vi "read station path config.vi"(8 "error in":errorcluster, 10 "station idx":i32, 11 "configuration file path in":path) -> (0 "error out":errorcluster, 2 "paths":T1={"Base Path"=path "", "system error log path"=path "", "Error Table Path"=path "", "Store errors log path"=path "", "data bytes log path"=path "", "network path"=path "C:/Labview Code/System/Error Table"}, 3 "configuration file path out":path)   [LabVIEW 2018]
uses:
  02.Type Def's/station paths.ctl
  05.UserVI's/file io/ini/type defs/ini file actions.ctl
  05.UserVI's/file io/ini/type defs/ini entry value.ctl
  05.UserVI's/file io/ini/type defs/ini entry types.ctl
  05.UserVI's/file io/ini/type defs/ini entry.ctl
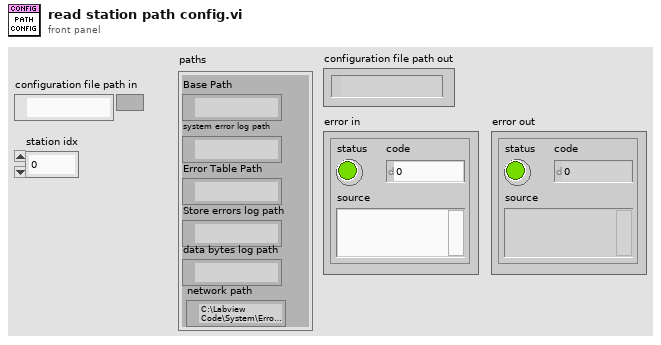
[diagram p1: front panel]
types:
  T1 = typedef "station paths.ctl" = cluster{"Base Path":path, "system error log path":path, "Error Table Path":path, "Store errors log path":path, "data bytes log path":path, "network path":path}
  T2 = typedef "ini entry value.ctl" = cluster{"Boolean":bool, "Dbl":dbl, "I32":i32, "Path":path, "String":string, "U32":u32}
  T3 = typedef "ini file actions.ctl" = enum16{"read ini", "write ini"}
  T4 = typedef "ini entry.ctl" = cluster{"section":string, "key":string, "type":T5, "default value":T2}
  T5 = typedef "ini entry types.ctl" = enum16{"Boolean", "Double", "I32", "Path", "String", "U32"}
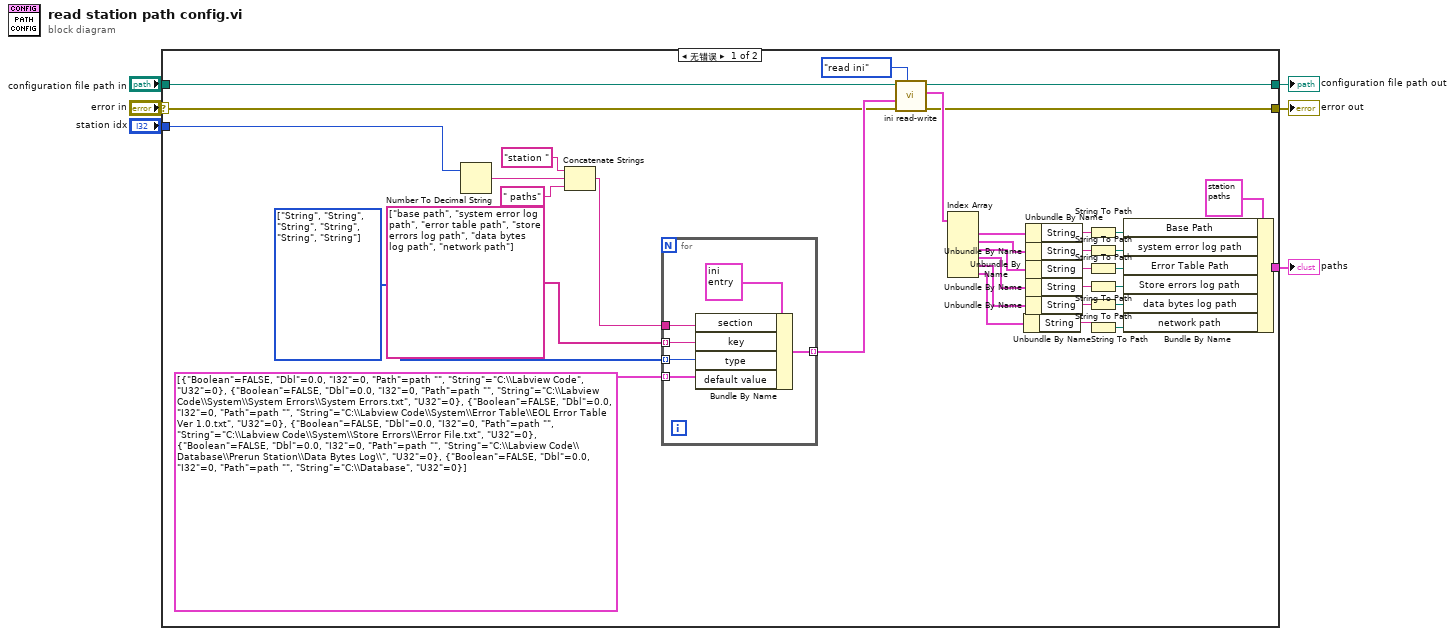
[diagram p0: block diagram]
diagram:
  n1 = case shown="无错误" "error in" {
    selector: "error in" -> [w11 w49]
    tunnel: [w41 _] -> w6
    tunnel: "configuration file path in" -> [w39 w48]
    tunnel: [w34 w48] -> w4
    tunnel: [w33 w49] -> w3
    tunnel: "station idx" -> [w31 _]
    frame No Error {
      w14 = T5[] [enum."String", enum."String", enum."String", enum."String", enum."String", enum."String"] items=["Boolean", "Double", "I32", "Path", "String", "U32"]
      n2 = Number To Decimal String(number=w31) -> (decimal integer string=w30:string)  [unwired: 1 in]
      n3 = Concatenate Strings("station ", w30, " paths" ("string")) -> (w29:string)
      n4 = for {
        tunnel: w29 -> [w46]
        tunnel: string[] ["base path", "system error log path", "error table path", "store errors log path", "data bytes log path", "network path"] -> [w45] mode=indexing
        tunnel: w14 -> [w44] mode=indexing
        tunnel: T2[] [{"Boolean"=FALSE, "Dbl"=0.0, "I32"=0, "Path"=path "", "String"="C:\\Labview Code", "U32"=0}, {"Boolean"=FALSE, "Dbl"=0.0, "I32"=0, "Path"=path "", "String"="C:\\Labview Code\\System\\System Errors\\System Errors.txt", "U32"=0}, {"Boolean"=FALSE, "Dbl"=0.0, "I32"=0, "Path"=path "", "String"="C:\\Labview Code\\System\\Error Table\\EOL Error Table Ver 1.0.txt", "U32"=0}, {"Boolean"=FALSE, "Dbl"=0.0, "I32"=0, "Path"=path "", "String"="C:\\Labview Code\\System\\Store Errors\\Error File.txt", "U32"=0}, {"Boolean"=FALSE, "Dbl"=0.0, "I32"=0, "Path"=path "", "String"="C:\\Labview Code\\Database\\Prerun Station\\Data Bytes Log\\", "U32"=0}, {"Boolean"=FALSE, "Dbl"=0.0, "I32"=0, "Path"=path "", "String"="C:\\Database", "U32"=0}] -> [w43] mode=indexing
        tunnel: [w42] -> w12 mode=indexing
        n5 = Bundle By Name(cluster=T4 {"section"="", "key"="", "type"=enum."Boolean", "default value"={"Boolean"=FALSE, "Dbl"=0.0, "I32"=0, "Path"=path "", "String"="", "U32"=0}}, "section"=w46, "key"=w45, "type"=w44, "default value"=w43) -> (w42:T4)
      }
      n6 = call "ini read-write.vi"("action"=ini_file_actions."read ini", "error in (no error)"=w11, "ini entry descriptors"=w12, "configuration file path"=w39) -> ("error out"=w33:errorcluster, "values out"=w37:T2[], "configuration file path out"=w34:path)  [unwired: 5 in]
      n7 = Index Array(array=w37) -> (element #1=w36:T2, element #2=w35:T2, element #3=w18:T2, element #4=w17:T2, element #5=w16:T2, element #6=w9:T2)  [unwired: 6 in]
      n8 = Unbundle By Name(w9) -> ("String"=w8:string)
      n9 = Unbundle By Name(w36) -> ("String"=w28:string)
      n10 = Unbundle By Name(w35) -> ("String"=w26:string)
      n11 = Unbundle By Name(w18) -> ("String"=w25:string)
      n12 = Unbundle By Name(w17) -> ("String"=w24:string)
      n13 = Unbundle By Name(w16) -> ("String"=w23:string)
      n14 = String To Path(string=w28) -> (path=w27:path)
      n15 = String To Path(string=w26) -> (path=w22:path)
      n16 = String To Path(string=w25) -> (path=w21:path)
      n17 = String To Path(string=w24) -> (path=w20:path)
      n18 = String To Path(string=w23) -> (path=w19:path)
      n19 = String To Path(string=w8) -> (path=w7:path)
      n20 = Bundle By Name(cluster=T1 {"Base Path"=path "", "system error log path"=path "", "Error Table Path"=path "C:/Labview Code/System/Error Table", "Store errors log path"=path "C:/Labview Code/System/Error Table", "data bytes log path"=path "C:/Labview Code/System/Error Table", "network path"=path ""} ("paths"), "Base Path"=w27, "system error log path"=w22, "Error Table Path"=w21, "Store errors log path"=w20, "data bytes log path"=w19, "network path"=w7) -> (w41:T1)
    }
    frame Error {
    }
  }
  "paths" <- w6
  "configuration file path out" <- w4
  "error out" <- w3
